vi "MCS_VGap_GapRecover.vi"() -> ()   [LabVIEW 2010]
panel:
  out "error out":errorcluster
  in  "Gap Change (um)":i32
  in  "?":bool
  out "Position 3 (um)":dbl
  out "Position 2 (um)":dbl
  out "Position 1 (um)":dbl
  in  "?":bool
  in  "System Locator":string
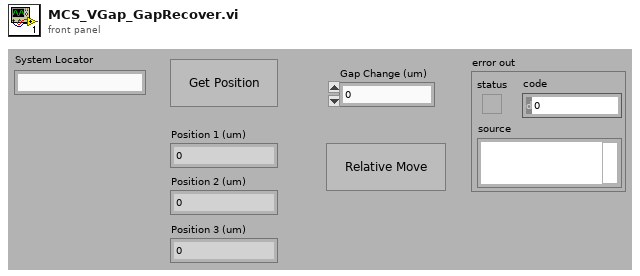
[diagram p1: front panel]
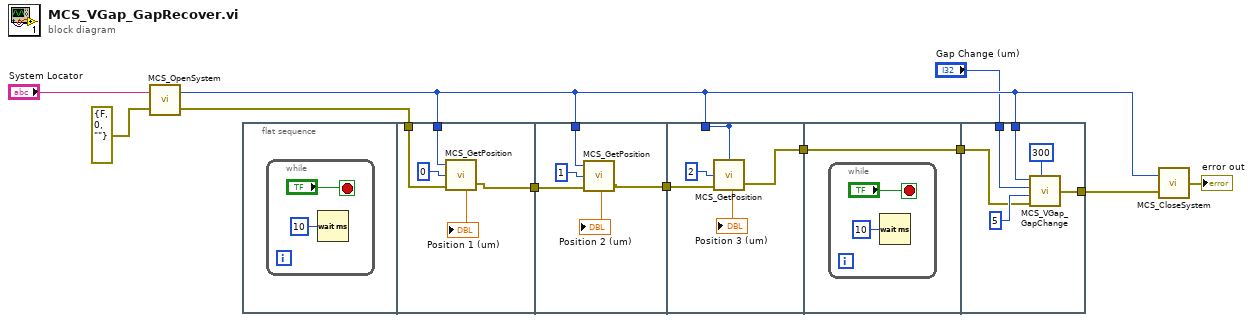
[diagram p0: block diagram]
diagram:
  n1 = call "MCS_OpenSystem.vi"("error in (no error)"=errorcluster {"status"=FALSE, "code"=0, "source"=""}, "MCS System Locator"="System Locator") -> ("error out"=w8:errorcluster, "System Index Out"=w9:u32)
  n2 = flat-sequence {
    tunnel: w8 -> [w16]
    tunnel: w9 -> [w15]
    tunnel: [w14] -> w5
    tunnel: w9 -> [w22]
    tunnel: w5 -> [w21]
    tunnel: [w19] -> w4
    tunnel: w4 -> [w27]
    tunnel: [w26] -> _
    tunnel: w9 -> [w26]
    tunnel: [w24] -> w3
    tunnel: w3 -> [w29]
    tunnel: [w29] -> w2
    tunnel: w2 -> [w33]
    tunnel: w9 -> [w36]
    tunnel: "Gap Change (um)" -> [w35]
    tunnel: [w32] -> w7
    frame #0 {
      n3 = while {
        stop <- "?" stop-if-true
        n4 = Wait (ms)(milliseconds to wait=u32 10) -> ()  [unwired: 1 out]
      }
    }
    frame #1 {
      n5 = call "MCS_GetPosition.vi"("error in (no error)"=w16, "Channel Index In"=u32 0, "System Index In"=w15) -> ("error out"=w14:errorcluster, "Position (um)"=→"Position 1 (um)":dbl)
    }
    frame #2 {
      n6 = call "MCS_GetPosition.vi"("error in (no error)"=w21, "Channel Index In"=u32 1, "System Index In"=w22) -> ("error out"=w19:errorcluster, "Position (um)"=→"Position 2 (um)":dbl)
    }
    frame #3 {
      n7 = call "MCS_GetPosition.vi"("error in (no error)"=w27, "Channel Index In"=u32 2, "System Index In"=w26) -> ("error out"=w24:errorcluster, "Position (um)"=→"Position 3 (um)":dbl)
    }
    frame #4 {
      n8 = while {
        stop <- "?" stop-if-true
        n9 = Wait (ms)(milliseconds to wait=u32 10) -> ()  [unwired: 1 out]
      }
    }
    frame #5 {
      n10 = call "MCS_VGap_GapChange.vi"("System Index In"=w36, "Gap Change (um)"=w35, "Step Change (um)"=5, "error in (no error)"=w33, "Stage Delay (ms)"=300) -> ("error out"=w32:errorcluster)
    }
  }
  n11 = call "MCS_CloseSystem.vi"("error in (no error)"=w7, "System Index In"=w9) -> ("error out"=→"error out":errorcluster)
